vi "Create Waveform Cluster (1D).vi"(1 "dx":dbl, 2 "Y":dbl[](array[numeric]), 4 "offset":dbl) -> (5 "waveform cluster":cluster{dbl, "dx":dbl, "Y":dbl[]})   [LabVIEW 2020]
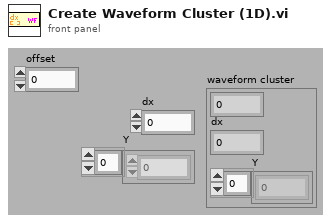
[diagram p1: front panel]
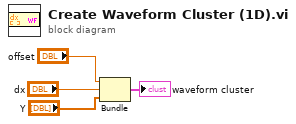
[diagram p0: block diagram]
diagram:
  n1 = Bundle("offset"="offset", "dx"="dx", "Y"="Y") -> (→"waveform cluster":cluster{"offset":dbl, "dx":dbl, "Y":dbl[]})  [unwired: 1 in]
